vi "RD device Open.vi"(8 "error in (no error)":errorcluster caption="错误输入（无错误）", 10 "ftHandle":u64, 11 "i":i32) -> (0 "error out":errorcluster caption="错误输出", 2 "ftHandle out":u64, 3 "function return":i32)   [LabVIEW 2018, in "InstrumentsPlayground.lvlib"]
doc: "CLIFFAPI int CliffdeviceOpen(int i,FT_HANDLE *ftHandle);"
uses:
  InstrumentsPlayground.lvlib
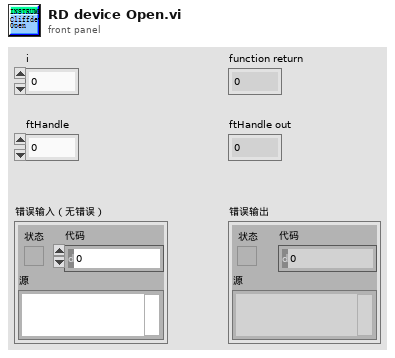
[diagram p1: front panel]
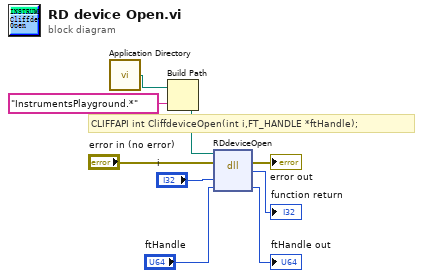
[diagram p0: block diagram]
diagram:
  # "CLIFFAPI int CliffdeviceOpen(int i,FT_HANDLE *ftHandle);"
  n1 = call <vilib>:"Application Directory.vi"() -> ("Application Directory"=w2:path)
  n2 = Build Path(base path=w2, name or relative path="InstrumentsPlayground.*" ("名称或相对路径")) -> (appended path=w1:path)
  n3 = dll-call lib="E:/work/YZCourse_Xtext/Cliff/API/LabVIEW lib/InstrumentsPlayground.*" fn="RDdeviceOpen"(path in=w1, error in="error in (no error)", "i"="i", "ftHandle"="ftHandle") -> (error out=→"error out":errorcluster, "返回类型"=→"function return":i32, "ftHandle"=→"ftHandle out":u32)  [unwired: 2 in, 1 out]
